vi "SendEth.vi"(4 "Msg":T1, 5 "conn ID":refnum<k5>) -> (1 "status":bool)   [LabVIEW 2010]
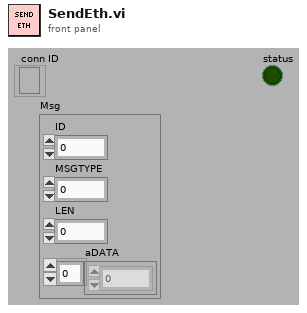
[diagram p1: front panel]
types:
  T1 = cluster{"ID":u32, "MSGTYPE":u8, "LEN":u8, "aDATA":u8[]}
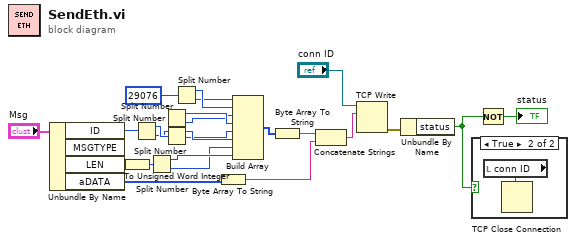
[diagram p0: block diagram]
diagram:
  n1 = Unbundle By Name("Msg") -> ("ID"=w13:u32, "LEN"=w6:u8, "aDATA"=w22:u8[])  [unwired: 1 out]
  n2 = To Unsigned Word Integer(number=w6) -> (unsigned 16bit integer=w5:u16)
  n3 = Split Number(x=w13) -> (hi(x)=w12:u16, lo(x)=w7:u16)
  n4 = Split Number(x=w5) -> (hi(x)=w4:u8, lo(x)=w3:u8)
  n5 = Split Number(x=w7) -> (hi(x)=w11:u8, lo(x)=w10:u8)
  n6 = Split Number(x=w12) -> (hi(x)=w9:u8, lo(x)=w8:u8)
  n7 = Split Number(x=u16 29076 ("element")) -> (hi(x)=w16:u8, lo(x)=w15:u8)
  n8 = Byte Array To String(unsigned byte array=w22) -> (string=w19:string)
  n9 = Build Array(w15, w16, w10, w11, w8, w9, w3, w4) -> (w21:u8[])
  n10 = Byte Array To String(unsigned byte array=w21) -> (string=w20:string)
  n11 = Concatenate Strings(w20, w19) -> (w18:string)
  n12 = TCP Write(connection ID="conn ID", data in=w18) -> (error out=w23:errorcluster)  [unwired: 2 in, 2 out]
  n13 = Unbundle By Name(w23) -> ("status"=w2:bool)
  n14 = case shown="True" w2 {
    frame False {
    }
    frame True {
      n15 = local read "conn ID"() -> (w25:refnum<k5>)
      n16 = TCP Close Connection(connection ID=w25) -> ()  [unwired: 2 in, 2 out]
    }
  }
  n17 = Not(x=w2) -> (.not. x?=→"status":bool)
